vi "test Connect Multiple.vi"(8 "error in (no error)":errorcluster, 11 "TestCase in":refnum<class "%DEVICE% Messaging Tests.lvclass">) -> (0 "error out":errorcluster, 3 "TestCase out":refnum<class "%DEVICE% Messaging Tests.lvclass">)   [LabVIEW 2017, in "%DEVICE% Messaging Tests.lvclass"]
uses:
  %DEVICE% Messaging Tests.lvclass
  Includes/CDMessaging.lvlibp/Switch/Switch Connect Message/Switch Connect Message.lvclass
  C:/Users/Admin/Documents/niveristand-routing-and-faulting-message-library/Includes/CDMessaging.lvlibp/Message/Abstract Message/Abstract Message.lvclass
  Support/Mock %DEVICE% Consumer.lvclass
  %DEVICE% Messaging Tests.lvclass/%DEVICE% Messaging Tests.ctl
  Support/Mock %DEVICE% Consumer.lvclass/Mock %DEVICE% Consumer.ctl
  Support/Read Connections.vi
  Includes/CDMessaging.lvlibp/Switch/Abstract Switch Consumer/Abstract Switch Consumer.lvclass
  C:/Users/Admin/Documents/niveristand-routing-and-faulting-message-library/Includes/CDMessaging.lvlibp/Consumer/Abstract Consumer/Abstract Consumer.lvclass
  Includes/CDMessaging.lvlibp/Producer/Abstract Producer/Abstract Producer.lvclass
  <vilib>/addons/_JKI Toolkits/VI Tester/TestCase.llb/TestCase.lvclass
  Includes/CDMessaging.lvlibp/Consumer/Abstract Consumer/Abstract Consumer.lvclass
  C:/Program Files (x86)/National Instruments/LabVIEW 2017/vi.lib/addons/_JKI Toolkits/VI Tester/TestCase.llb/TestCase.lvclass
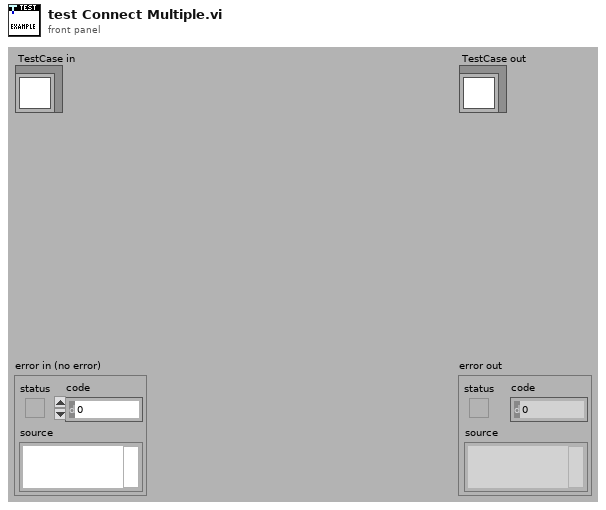
[diagram p1: front panel]
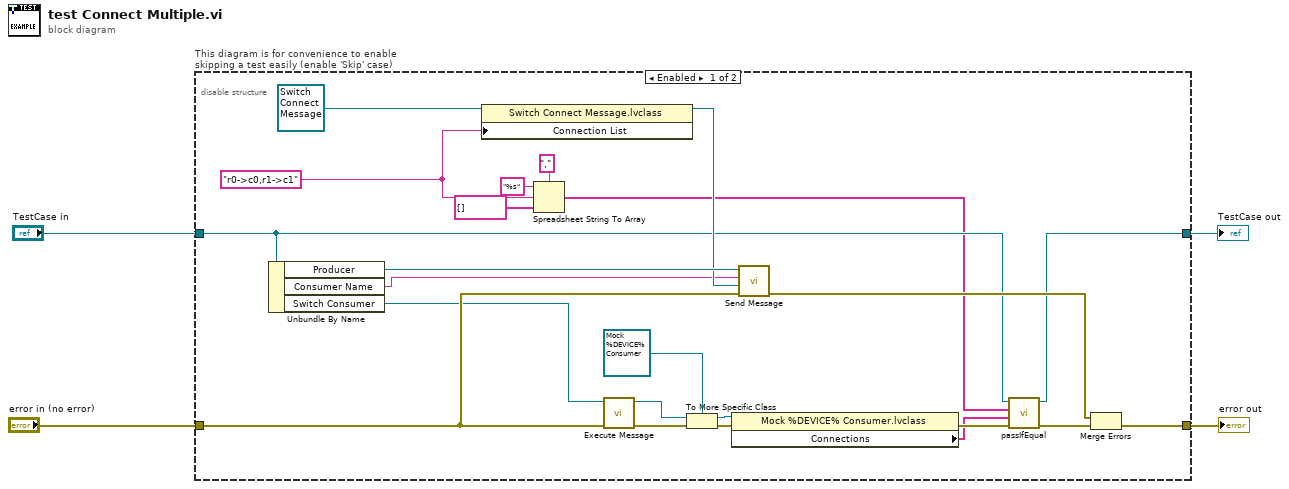
[diagram p0: block diagram]
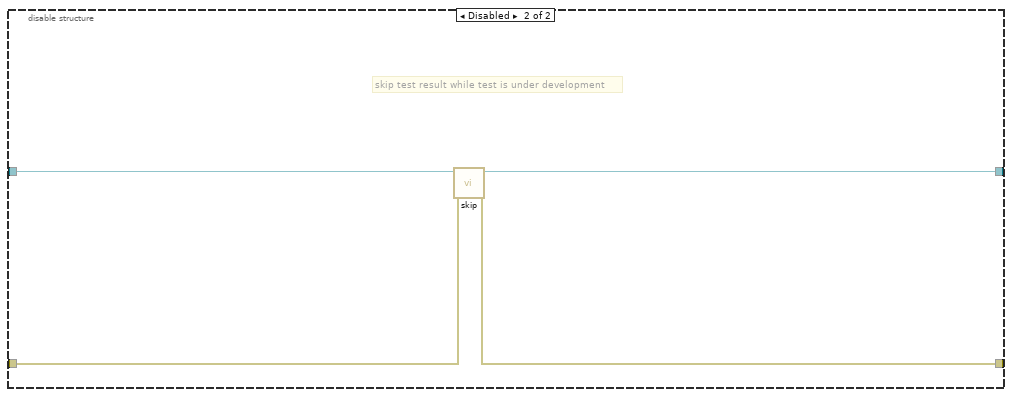
[diagram p2: hidden frame]
diagram:
  n1 = disable-structure "This diagram is for convenience to enable skipping a test easily (enable 'Skip' case)" shown="Enabled" {
    disable-tunnel: "TestCase in" -> [w12 w31]
    disable-tunnel: [w11 w29] -> w1
    disable-tunnel: [w20 w30] -> w3
    disable-tunnel: "error in (no error)" -> [w23 w28]
    frame Enabled {
      w9 = "r0->c0,r1->c1"
      n2 = Unbundle By Name(w12) -> ("Producer"=w26:refnum<class "Abstract Producer.lvclass">, "Consumer Name"=w24:string, "Switch Consumer"=w22:refnum<class "Abstract Switch Consumer.lvclass">)
      n3 = property class="Switch Connect Message.lvclass"(reference=refnum<class "Switch Connect Message.lvclass"> refnum ("CDMessaging.lvlibp:Switch Connect Message.lvclass"), "Connection List"=w9) -> (reference out=w25:refnum<class "Switch Connect Message.lvclass">)  [unwired: 1 in, 1 out]
      n4 = Spreadsheet String To Array(delimiter (Tab)=",", format string="%s", spreadsheet string=w9, array type (2D Dbl)=string[] []) -> (array=w8:string[])
      n5 = call "Execute Message.vi"("error in (no error)"=w23, "Abstract Consumer in"=w22) -> ("error out"=w19:errorcluster, "Abstract Consumer out"=w17:refnum<class "Abstract Consumer.lvclass">)  [unwired: 6 in, 2 out]
      n6 = To More Specific Class(target class=refnum<class "Mock %DEVICE% Consumer.lvclass"> refnum ("Mock NI-SWITCH Consumer.lvclass"), reference=w17, error in=w19) -> (specific class reference=w14:refnum<class "Mock %DEVICE% Consumer.lvclass">, error out=w16:errorcluster)
      n7 = property class="Mock %DEVICE% Consumer.lvclass"(reference=w14, error in=w16) -> (error out=w15:errorcluster, "Connections"=w10:string[])  [unwired: 1 out]
      n8 = call-dynamic "Send Message.vi"("error in (no error)"=w23, "Message in"=w25, "Consumer in"=w24, "Abstract Producer in"=w26) -> ("error out"=w21:errorcluster)  [unwired: 4 in, 3 out]
      n9 = call-dynamic "passIfEqual.vi"("error in (no error)"=w15, "y"=w10, "x"=w8, "TestCase in"=w12) -> ("error out"=w13:errorcluster, "TestCase out"=w11:refnum<class "%DEVICE% Messaging Tests.lvclass">)  [unwired: 6 in]
      n10 = Merge Errors(w21, w13) -> (w20:errorcluster)
    }
    frame Disabled {
      # "skip test result while test is under development"
      n11 = call <vilib>:"skip.vi"("error in (no error)"=w28, "TestCase in"=w31) -> ("error out"=w30:errorcluster, "TestCase out"=w29:refnum<class "%DEVICE% Messaging Tests.lvclass">)  [unwired: 8 in]
    }
  }
  "error out" <- w3
  "TestCase out" <- w1
